vi "Config - Insert.vi"(8 "error in (no error)":errorcluster, 10 "Inserted Data":T1, 11 "Config Records":T1[](array[typedef])) -> (0 "error out":errorcluster, 3 "Config Records":T1[](array[typedef]))   [LabVIEW 2017]
doc: "Provide insert operation for configuration database process.\n[Covers: SD5]"
uses:
  Controls/Config Record.ctl
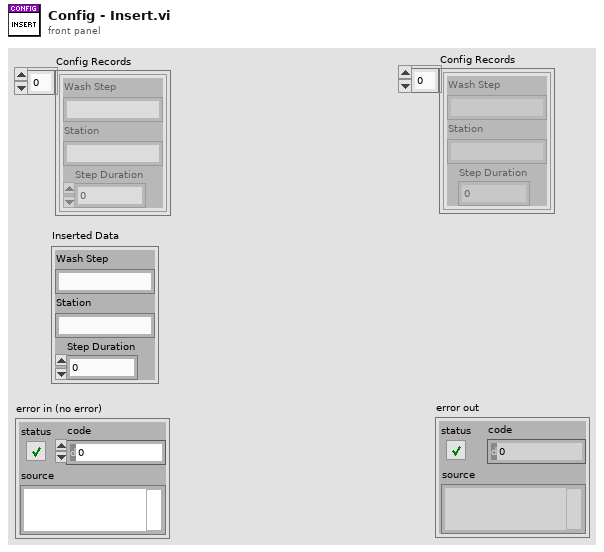
[diagram p1: front panel]
types:
  T1 = typedef "Config Record.ctl" = cluster{"Wash Step":string, "Station":string, "Step Duration":u32}
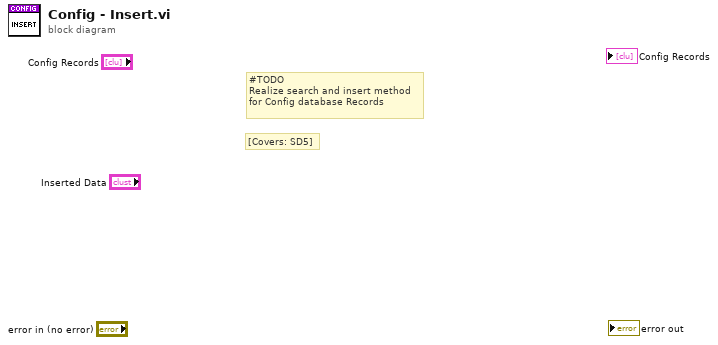
[diagram p0: block diagram]
diagram:
  # "[Covers: SD5]"
  # "#TODO\nRealize search and insert method\nfor Config database Records"
